vi "Program_Active_Client.vi"(3 "Mode":enum16{"Program Active", "Traverse Level State"}(ring), 4 "Time till next contact (Sec)":dbl=60.0 min=0.0, 5 "Traverse level State":T1) -> ()   [LabVIEW 2010]
doc: "This is an example of using features of the VI Server as a client. It shows how you might browse from one or more applications that may be exporting data from one or more data stations. \n\nThe example shows how to query a server for its list of exported VIs, how to get references to the VIs, and how call them with the Call By Reference function."
uses:
  Sub VIs/ADAM Controls/Traverse_Level_State.ctl
  Anemometry/Anemometry Sub Vis/Globals/Meas_global.vi
  Anemometry/Anemometry Sub Vis/Globals/Preference_global.vi
  Anemometry/Anemometry Sub Vis/Globals/Dynamic_call_global.ph.vi
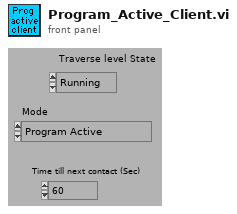
[diagram p1: front panel]
types:
  T1 = typedef "Traverse_Level_State.ctl" = enum16{"Running", "Complete"}
  T2 = typedef "Server_Comms.ctl" = enum16{"Server Link Healthy", "Do Not Link To Server"}
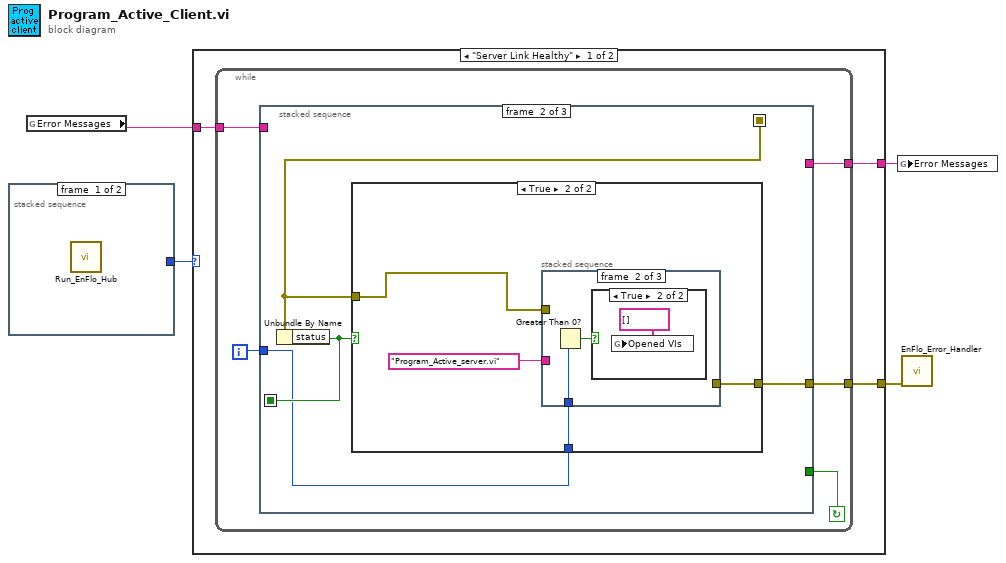
[diagram p0: block diagram]
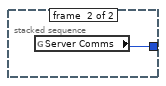
[diagram p2: hidden frame]
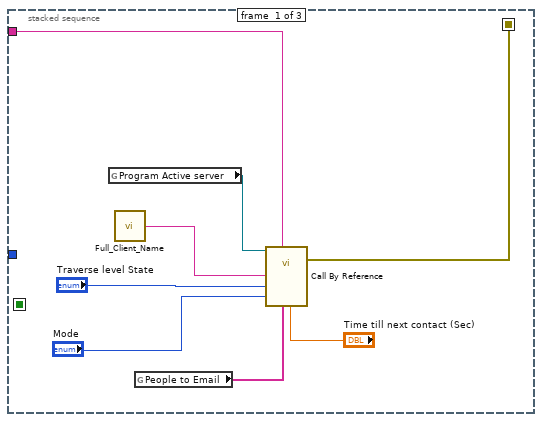
[diagram p3: hidden frame]
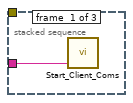
[diagram p5: hidden frame]
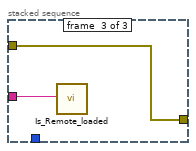
[diagram p7: hidden frame]
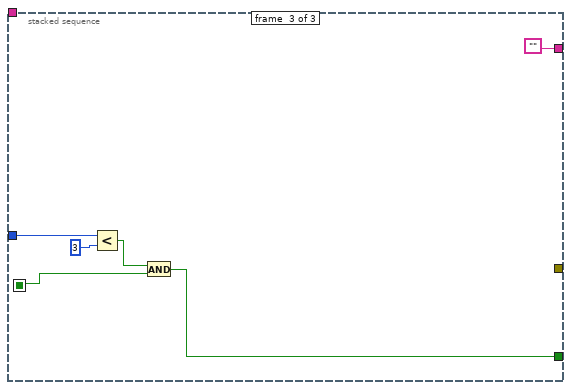
[diagram p8: hidden frame]
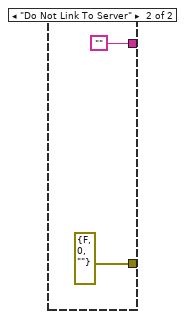
[diagram p9: hidden frame]
diagram:
  n1 = stacked-sequence {
    tunnel: [_ w5] -> w1
    frame #0 {
      n2 = call "Run_EnFlo_Hub.vi"() -> ()  [unwired: 8 out]
    }
    frame #1 {
      n3 = global read "Preference_global.vi" "Server Comms"() -> (w5:T2)
    }
  }
  n4 = global read "Meas_global.vi" "Error Messages"() -> (w3:string)
  n5 = case shown="\"Server Link Healthy\"" w1 {
    tunnel: [w8 errorcluster {"status"=FALSE, "code"=0, "source"=""} ("error in (no error)")] -> w4
    tunnel: w3 -> [w7 _]
    tunnel: [w6 ""] -> w2
    frame "Server Link Healthy" {
      n6 = while {
        tunnel: [w9] -> w6
        tunnel: w7 -> [w10]
        tunnel: [w11] -> w8
        i -> [w13]
        stop <- w12 continue-if-true
        n7 = stacked-sequence {
          seq-local: [w21 _ _] -> [_ w24 _]
          seq-local: [_ w25 _] -> [_ _ w39]
          tunnel: w13 -> [_ w23 w40]
          tunnel: [_ _ w38] -> w12
          tunnel: [_ w22 _] -> w11
          tunnel: w10 -> [w16 _ _]
          tunnel: [_ _ ""] -> w9
          frame #0 {
            n8 = global read "Dynamic_call_global.ph.vi" "Program Active server"() -> (w15:refnum<vi>)
            n9 = call "Full_Client_Name.vi"() -> ("Client Name"=w17:string)
            n10 = global read "Meas_global.vi" "People to Email"() -> (w18:string[])
            n11 = call-by-ref "?"(reference=w15, "Client Name"=w17, "Client Messages"=w16, "Traverse level State"="Traverse level State", "Mode"="Mode", "People to Email"=w18, "Time till next contact (Sec)"="Time till next contact (Sec)") -> (error out=w21:errorcluster)  [unwired: 6 in, 1 out]
          }
          frame #1 {
            n12 = Unbundle By Name(w24) -> ("status"=w25:bool)
            n13 = case shown="True" w25 {
              tunnel: w24 -> [w26 w29]
              tunnel: w23 -> [_ w30]
              tunnel: [w26 w28] -> w22
              frame False {
              }
              frame True {
                n14 = stacked-sequence {
                  tunnel: "Program_Active_server.vi" -> [w31 _ w36]
                  tunnel: w30 -> [_ w33 _]
                  tunnel: w29 -> [_ _ w35]
                  tunnel: [_ _ w35] -> w28
                  frame #0 {
                    n15 = call "Start_Client_Coms.vi"("VI name to run on server"=w31) -> ()  [unwired: 1 in, 4 out]
                  }
                  frame #1 {
                    n16 = Greater Than 0?(x=w33) -> (x > 0?=w32:bool)
                    n17 = case shown="True" w32 {
                      frame False {
                      }
                      frame True {
                        n18 = global write "Dynamic_call_global.ph.vi" "Opened VIs"(string[] [] ("Opened VIs")) -> ()
                      }
                    }
                  }
                  frame #2 {
                    n19 = call "Is_Remote_loaded.vi"("Sub VI to call"=w36) -> ()
                  }
                }
              }
            }
          }
          frame #2 {
            n20 = Less?(x=w40, y=3) -> (x < y?=w42:bool)
            n21 = And(x=w42, y=w39) -> (x .and. y?=w38:bool)
          }
        }
      }
    }
    frame "Do Not Link To Server" {
    }
  }
  n22 = global write "Meas_global.vi" "Error Messages"(w2) -> ()
  n23 = call "EnFlo_Error_Handler.vi"("error in (no error)"=w4) -> ()  [unwired: 2 in, 3 out]
